vi "Read Temperature.vi"(0 "Session Handle in":T1, 11 "error in (no error)":errorcluster) -> (4 "Session Handle out":T1, 6 "Temperature":dbl, 8 "Success?":bool, 10 "Error Code":string, 15 "error out":errorcluster)   [LabVIEW 2015, in "PAS.lvclass"]
uses:
  PAS.lvclass
  Typedefs/Session Handle.ctl
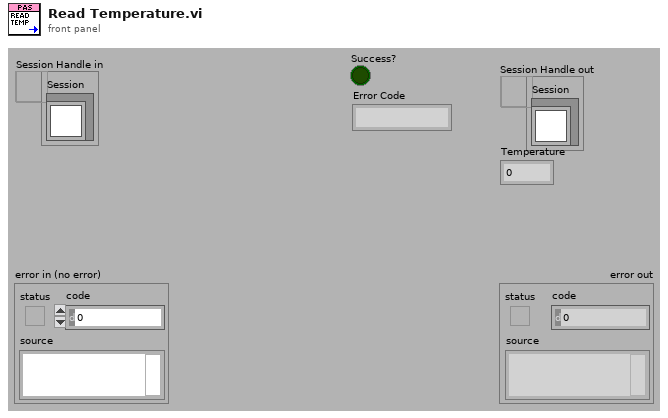
[diagram p1: front panel]
types:
  T1 = typedef "PAS.lvclass/Session Handle.ctl" = refnum<data-value>
  T2 = typedef "XNET Frame CAN.ctl" = cluster{"timestamp":timestamp, "payload":u8[], "identifier":u32, "type":T3, "extended?":bool, "echo?":bool}
  T3 = typedef "XNET Frame Type CAN.ctl" = u8
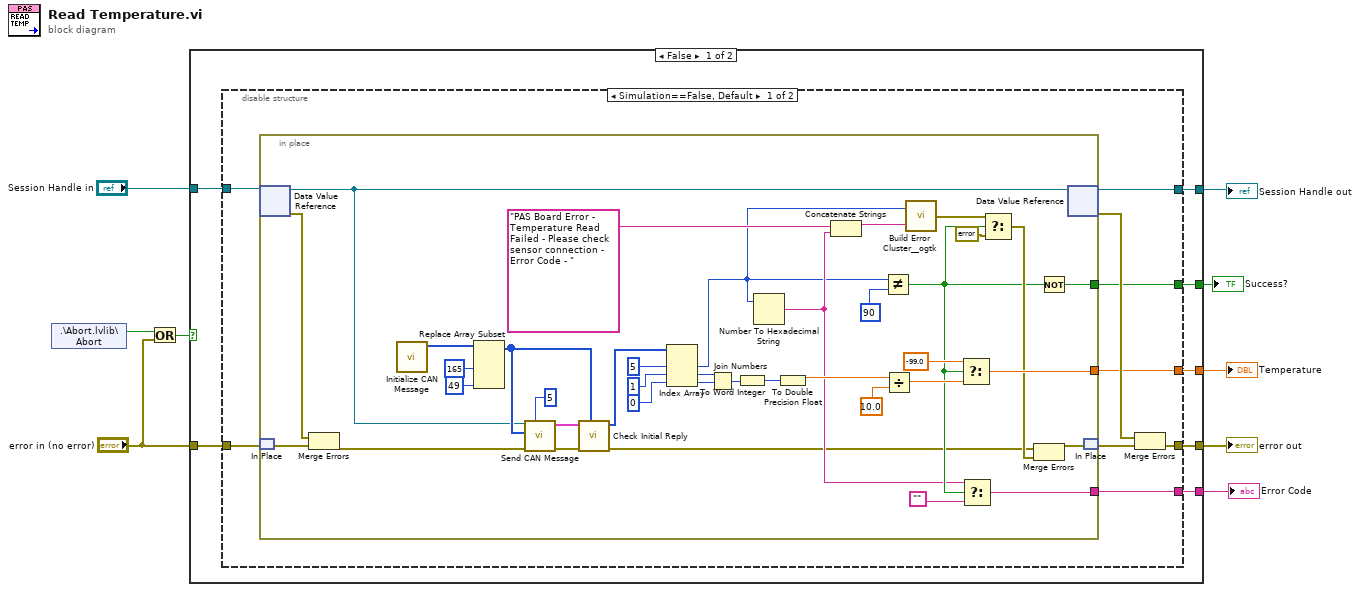
[diagram p0: block diagram]
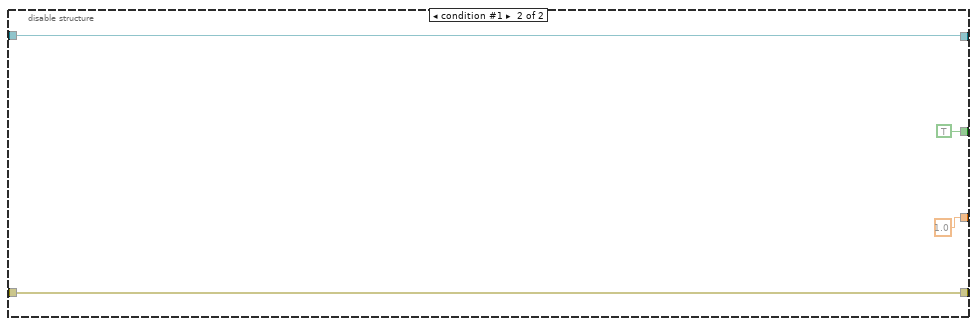
[diagram p2: hidden frame]
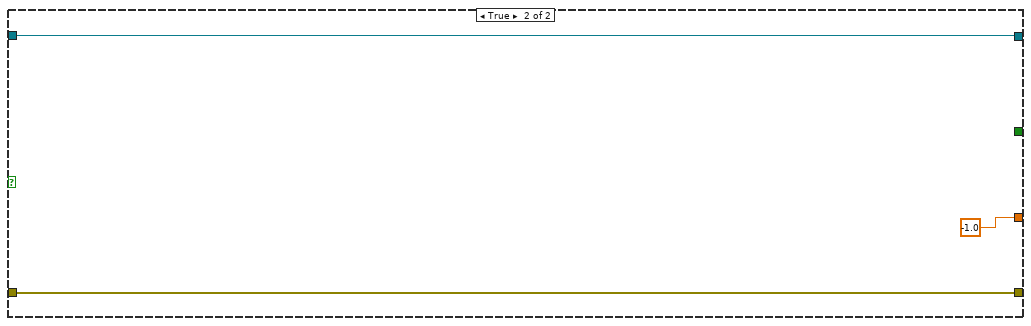
[diagram p3: hidden frame]
diagram:
  n1 = shared-variable ".\\Abort.lvlib\\Abort"() -> (w6:bool)  [unwired: 1 in, 1 out]
  n2 = Or(x=w6, y="error in (no error)") -> (x .or. y?=w4:bool)
  n3 = case shown="False" w4 {
    tunnel: [w16 w70] -> w8
    tunnel: [w15 w69] -> w7
    tunnel: "Session Handle in" -> [w14 w70]
    tunnel: "error in (no error)" -> [w13 w69]
    tunnel: [w12 -1.0] -> w3
    tunnel: [w11 _] -> w2
    tunnel: [w10 _] -> w1
    frame False {
      n4 = disable-structure shown="Simulation==False, Default" {
        disable-tunnel: [w25 w67] -> w16
        disable-tunnel: [w22 w66] -> w15
        disable-tunnel: w14 -> [w21 w67]
        disable-tunnel: w13 -> [w20 w66]
        disable-tunnel: [w19 1.0] -> w12
        disable-tunnel: [w18 TRUE] -> w11
        disable-tunnel: [w17 _] -> w10
        frame condition #0 (active) {
          n5 = in-place {
            in-place-border: [w38] -> w19
            in-place-border: [w49] -> w18
            in-place-border: [w29] -> w17
            n6 = in-place-dvr #1(w21) -> (w54:refnum<class "PAS.lvclass">, w59:errorcluster)
            n7 = in-place-match #2(w20) -> (w58:errorcluster)
            n8 = Merge Errors(w59, w58) -> (w53:errorcluster)
            n9 = call "Initialize CAN Message.vi"() -> ("Initial Payload"=w61:u8[])  [unwired: 11 in]
            n10 = Replace Array Subset(array=w61, new element #1=u8 165 ("new element/subarray"), new element #2=u8 49 ("new element/subarray")) -> (w57:u8[])  [unwired: 2 in]
            n11 = call "Send CAN Message.vi"("Number of Retries"=5, "error in (no error)"=w53, "payload"=w57, "Pas In"=w54) -> ("error out"=w28:errorcluster, "Reply"=w55:T2[])  [unwired: 5 in, 1 out]
            n12 = call "Check Initial Reply.vi"("Write Message"=w57, "error in (no error)"=w28, "Reply"=w55) -> ("error out"=w27:errorcluster, "Data Packet"=w60:u8[])  [unwired: 5 in, 2 out]
            n13 = Index Array(array=w60, index #1=5 ("index"), index #2=1 ("index"), index #3=0 ("index")) -> (element #1=w26:u8, element #2=w45:u8, element #3=w44:u8)
            n14 = Join Numbers(hi=w45, lo=w44) -> ((hi.lo)=w43:u16)
            n15 = To Word Integer(number=w43) -> (16bit integer=w46:i16)
            n16 = Number To Hexadecimal String(2:w26) -> (0:w30:string)  [unwired: 1 in]
            n17 = To Double Precision Float(number=w46) -> (double precision float=w40:dbl)
            n18 = Concatenate Strings("PAS Board Error - Temperature Read Failed - Please check sensor connection -  Error Code - " ("string"), w30) -> (w52:string)
            n19 = Not Equal?(x=w26, y=u8 90 ("new element/subarray")) -> (x != y?=w31:bool)
            n20 = Divide(x=w40, y=10.0) -> (x/y=w35:dbl)
            n21 = call <userlib>:"Build Error Cluster__ogtk.vi"("String to Prepend to source (\"\")"=w52, "code"=w26) -> ("error out"=w42:errorcluster)
            n22 = Select(t=-99.0, s=w31, f=w35) -> (s? t:f=w38:dbl)
            n23 = Select(t=w30, s=w31, f="") -> (s? t:f=w29:string)
            n24 = Select(t=w42, s=w31, f=errorcluster {"status"=FALSE, "code"=0, "source"=""}) -> (s? t:f=w33:errorcluster)
            n25 = Merge Errors(w27, w33) -> (w62:errorcluster)
            n26 = Not(x=w31) -> (.not. x?=w49:bool)
            n27 = in-place-dvr #1(w54) -> (w25:T1, w23:errorcluster)
            n28 = in-place-match #2(w62) -> (w24:errorcluster)
          }
          n29 = Merge Errors(w23, w24) -> (w22:errorcluster)
        }
        frame condition #1 {
        }
      }
    }
    frame True {
    }
  }
  "Session Handle out" <- w8
  "error out" <- w7
  "Temperature" <- w3
  "Success?" <- w2
  "Error Code" <- w1
